vi "Copy.vi"(5 "XRef":refnum<vi>, 6 "State In":T1={"Output Type"=variant(dbl 0.0), "Name"="", "Input Type"=variant, "Constant Types"=[], "Error"={"status"=FALSE, "code"=0, "source"=""}, "Path"=path "", "Names"=[]}) -> (0 "Reply":string[](array[string]), 2 "State Out":T1={"Output Type"=variant(dbl 0.0), "Name"="", "Input Type"=variant, "Constant Types"=[], "Error"={"status"=FALSE, "code"=0, "source"=""}, "Path"=path "", "Names"=[]})   [LabVIEW 2015, in "Create-Signals.xnode"]
doc: "This ability VI is called by LabVIEW after the user copies an XNode. State In is the same as the original XNode's state. The generated code is copied from the old XNode and will not be regenerated unless you return the GenerateCode reply.\n\nDefault behavior: Produce an exact copy of the original XNode without regenerating the code.\n\nThis ability does not provide UI and OS messages are not handled.\n\nSee also: Initialize"
uses:
  Create-Signals.xnode
  State.ctl
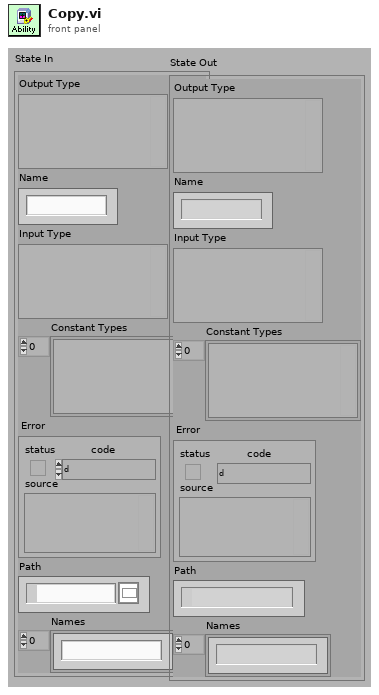
[diagram p1: front panel]
types:
  T1 = typedef "Create-Signals.xnode/State.ctl" = cluster{"Output Type":variant, "Name":string, "Input Type":variant, "Constant Types":variant[], "Error":errorcluster, "Path":path, "Names":string[]}
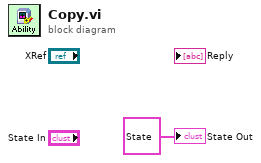
[diagram p0: block diagram]
diagram:
  "State Out" <- T1 {"Output Type"=variant, "Name"="", "Input Type"=variant, "Constant Types"=[], "Error"={"status"=FALSE, "code"=0, "source"=""}, "Path"=path "", "Names"=[]} ("State")
